vi "Configure TDMS.vi"(8 "error in (no error)":errorcluster, 11 "DataLogger in":refnum<class "DataLogger.lvclass">) -> (0 "error out":errorcluster, 3 "DataLogger out":refnum<class "DataLogger.lvclass">)   [LabVIEW 2020, in "Volatus.lvlib" / "DataLogger.lvclass"]
uses:
  DataLogger.lvclass
  C:/dev/lv20CE/relink/lv-volatus/Volatus/DataHandlerTask/DataHandlerTask.lvclass
  DataHandlerTask/DataHandlerTask.lvclass/DataHandlerTask.ctl
  DataLogger.lvclass/DataLogger.ctl
  DataHandlerTask/DataHandlerTask.lvclass
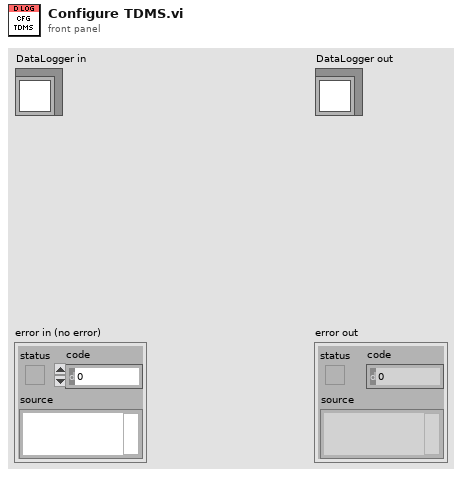
[diagram p1: front panel]
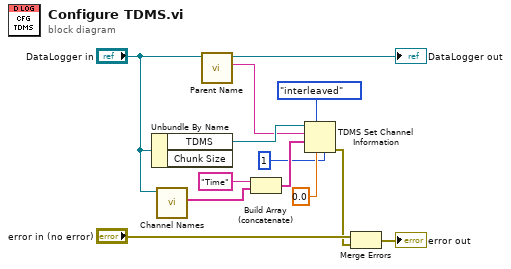
[diagram p0: block diagram]
diagram:
  n1 = Unbundle By Name("DataLogger in") -> ("TDMS"=w9:refnum<k34>)  [unwired: 1 out]
  n2 = call "Channel Names.vi"("DataHandlerTask in"="DataLogger in") -> ("Channel Names"=w3:string[])  [unwired: 8 in, 2 out]
  n3 = call "Parent Name.vi"("DataHandlerTask in"="DataLogger in") -> ("Parent Name"=w4:string, "DataHandlerTask out"=→"DataLogger out":refnum<class "DataLogger.lvclass">)  [unwired: 8 in, 1 out]
  n4 = Build Array (concatenate)("Time", w3) -> (w11:string[])
  n5 = TDMS Set Channel Information(4:u32 1 ("samples per channel"), 6:0.0, 7:enum16{"non-interleaved", "interleaved"}."interleaved" ("data layout (0:non-interleaved)"), 9:w11, 10:w4, 11:w9) -> (0:w6:errorcluster)  [unwired: 1 in, 1 out]
  n6 = Merge Errors("error in (no error)", w6) -> (→"error out":errorcluster)
